vi "getDeviceClockChannelRf.vi"(8 "error in (no error)":errorcluster, 10 "device":refnum<class "device.lvclass">, 11 "deviceDataBase in":refnum<class "deviceDataBase.lvclass">) -> (0 "error out":errorcluster, 1 "isClock":bool, 2 "timingChannel":refnum<class "Channel.lvclass">, 3 "deviceDataBase out":refnum<class "deviceDataBase.lvclass">, 4 "noChannel":bool)   [LabVIEW 2009, in "Tools.lvlib" / "DatabaseHelpers.lvlib" / "deviceDataBase.lvclass"]
uses:
  deviceDataBase.lvclass
  Database Objects/Channel/Channel.lvclass
  Database Objects/device/device.lvclass
  Database Objects/ChannelArray/ChannelArray.lvclass
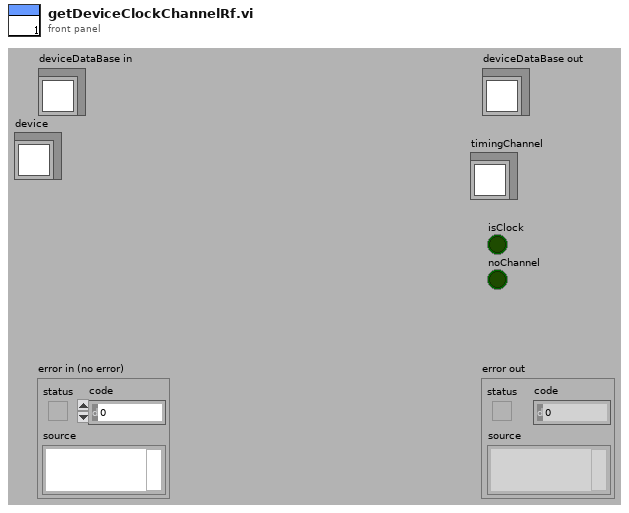
[diagram p1: front panel]
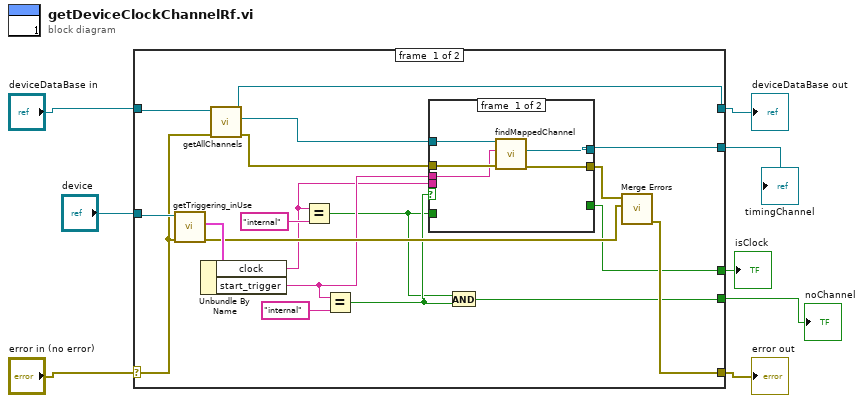
[diagram p0: block diagram]
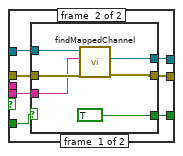
[diagram p2: hidden frame]
diagram:
  n1 = case shown="No Error" "error in (no error)" {
    selector: "error in (no error)" -> [w22 w48]
    tunnel: [w19 w48] -> w6
    tunnel: [w21 w47] -> w5
    tunnel: "deviceDataBase in" -> [w25 w47]
    tunnel: "device" -> [w27 _]
    tunnel: [w20 _] -> w4
    tunnel: [w12 _] -> w2
    tunnel: [w9 _] -> w1
    frame #0 {
      n2 = call "getTriggering_inUse.vi"("error in (no error)"=w22, "device.lvclass in"=w27) -> ("error out"=w16:errorcluster, "triggering_inUse"=w26:cluster{"start_trigger":string, "clock":string})  [unwired: 7 in, 1 out]
      n3 = Unbundle By Name(w26) -> ("clock"=w13:string, "start_trigger"=w15:string)
      n4 = call "getAllChannels.vi"("error in (no error)"=w22, "deviceDataBase in"=w25) -> ("error out"=w23:errorcluster, "ChannelArray.lvclass"=w24:refnum<class "ChannelArray.lvclass">, "deviceDataBase out"=w21:refnum<class "deviceDataBase.lvclass">)  [unwired: 7 in]
      n5 = Equal?(x=w13, y="internal") -> (x = y?=w10:bool)
      n6 = Equal?(x=w15, y="internal") -> (x = y?=w11:bool)
      n7 = case shown="True" w11 {
        tunnel: w24 -> [w32 w34]
        tunnel: w23 -> [w31 w37]
        tunnel: [w30 w35] -> w20
        tunnel: w15 -> [w28 _]
        tunnel: [w29 w36] -> w17
        tunnel: w10 -> [_ w39]
        tunnel: w13 -> [_ w38]
        tunnel: [_ w33] -> w12
        frame #0 {
          n8 = call "findMappedChannel.vi"("error in (no error)"=w31, "name of mappedTo channel"=w28, "ChannelArray in"=w32) -> ("error out"=w29:errorcluster, "Channel"=w30:refnum<class "Channel.lvclass">)  [unwired: 6 in, 1 out]
        }
        frame #1 {
          n9 = case shown="False" w39 {
            tunnel: w38 -> [w41 _]
            tunnel: w37 -> [w45 w46]
            tunnel: [w44 w46] -> w36
            tunnel: [w43 _] -> w35
            tunnel: w34 -> [w42 _]
            tunnel: [TRUE _] -> w33
            frame #0 {
              n10 = call "findMappedChannel.vi"("error in (no error)"=w45, "name of mappedTo channel"=w41, "ChannelArray in"=w42) -> ("error out"=w44:errorcluster, "Channel"=w43:refnum<class "Channel.lvclass">)  [unwired: 6 in, 1 out]
            }
            frame #1 {
            }
          }
        }
      }
      n11 = And(x=w10, y=w11) -> (x .and. y?=w9:bool)
      n12 = call <vilib>:"Merge Errors.vi"("error in 2 (no error)"=w16, "error in 1 (no error)"=w17) -> ("error out"=w19:errorcluster)  [unwired: 5 in]
    }
    frame #1 {
    }
  }
  "error out" <- w6
  "deviceDataBase out" <- w5
  "timingChannel" <- w4
  "isClock" <- w2
  "noChannel" <- w1
